vi "CSM - Replace Substitution Marks in States.vi"(5 "States with Replace Token":string, 7 "<param>":string, 9 "<target>":string, 11 "<other>":string, 12 "<1>":string, 13 "<2>":string) -> (6 "States":string)   [LabVIEW 2014, in "Communicable State Machine.lvlib"]
uses:
  Communicable State Machine.lvlib
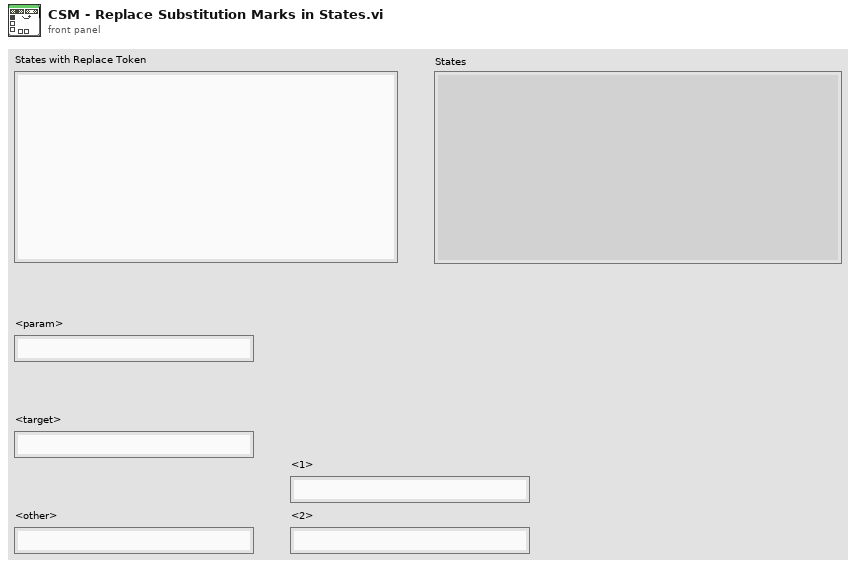
[diagram p1: front panel]
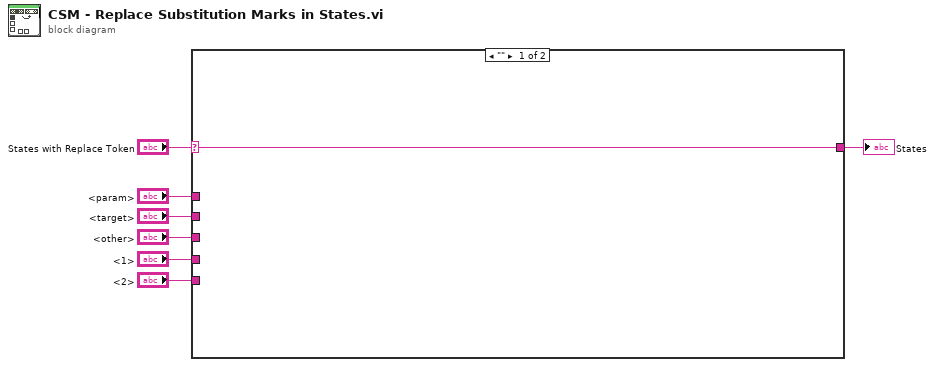
[diagram p0: block diagram]
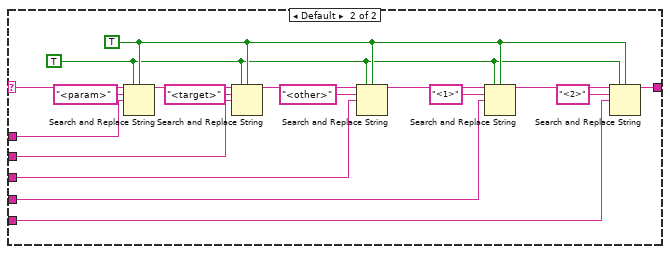
[diagram p2: hidden frame]
diagram:
  n1 = case shown="\"\"" "States with Replace Token" {
    selector: "States with Replace Token" -> [w8 w26]
    tunnel: "<param>" -> [_ w25]
    tunnel: "<target>" -> [_ w24]
    tunnel: "<other>" -> [_ w23]
    tunnel: [w8 w13] -> w6
    tunnel: "<2>" -> [_ w10]
    tunnel: "<1>" -> [_ w9]
    frame "" {
    }
    frame Default {
      w12 = TRUE ("ignore case? (F)")
      w11 = TRUE ("replace all? (F)")
      n2 = Search and Replace String(replace all?=w11, case sensitive?=w12, input string=w26, search string="<param>", replace string=w25) -> (result string=w22:string)  [unwired: 3 in, 3 out]
      n3 = Search and Replace String(replace all?=w11, case sensitive?=w12, input string=w22, search string="<target>", replace string=w24) -> (result string=w21:string)  [unwired: 3 in, 3 out]
      n4 = Search and Replace String(replace all?=w11, case sensitive?=w12, input string=w21, search string="<other>", replace string=w23) -> (result string=w14:string)  [unwired: 3 in, 3 out]
      n5 = Search and Replace String(replace all?=w11, case sensitive?=w12, input string=w14, search string="<1>", replace string=w9) -> (result string=w15:string)  [unwired: 3 in, 3 out]
      n6 = Search and Replace String(replace all?=w11, case sensitive?=w12, input string=w15, search string="<2>", replace string=w10) -> (result string=w13:string)  [unwired: 3 in, 3 out]
    }
  }
  "States" <- w6
